vi "Show Vi Panel.vi"(8 "error in (no error)":errorcluster, 11 "Vi Ref":refnum<vi>) -> (0 "error out":errorcluster)   [LabVIEW 2014, in "Chart Module.lvlib"]
uses:
  Chart Module.lvlib
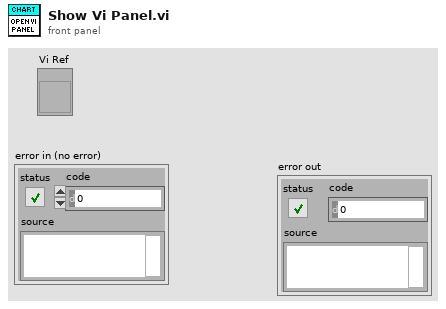
[diagram p1: front panel]
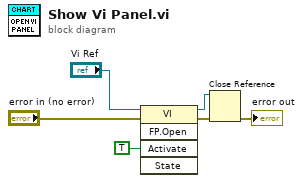
[diagram p0: block diagram]
diagram:
  n1 = invoke class="VI" method="FP.Open"(reference="Vi Ref", error in="error in (no error)", "Activate"=TRUE ("Activate?")) -> (reference out=w3:refnum<vi>, error out=w1:errorcluster)  [unwired: 2 in, 3 out]
  n2 = Close Reference(reference=w3, error in (no error)=w1) -> (error out=→"error out":errorcluster)
